vi "Get Ingredients.vi"(8 "error in (no error)":errorcluster, 11 "Wood in":refnum<class "Wood.lvclass">) -> (0 "error out":errorcluster, 2 "Ingredients":T1[](array[typedef]), 3 "Wood out":refnum<class "Wood.lvclass">)   [LabVIEW 2020, in "Wood.lvclass"]
uses:
  Wood.lvclass
  Item/Ingredient.ctl
  Item/Item.lvclass
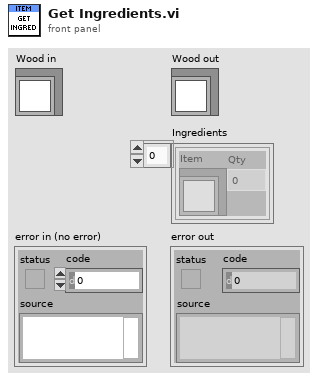
[diagram p1: front panel]
types:
  T1 = typedef "Item.lvclass/Ingredient.ctl" = cluster{"Item":refnum<class "Item.lvclass">, "Qty":dbl}
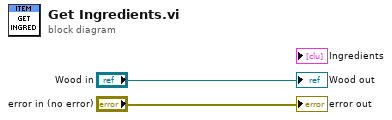
[diagram p0: block diagram]
diagram:
  "error out" <- "error in (no error)"
  "Wood out" <- "Wood in"
